vi "ErrorDescription.vi"(1 "AxisReadValues.AxisErrorCode":i16) -> (0 "ErrorDescription":string)   [LabVIEW 2020, in "SMCD14_lib.lvlib"]
uses:
  SMCD14_lib.lvlib
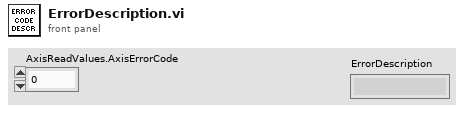
[diagram p1: front panel]
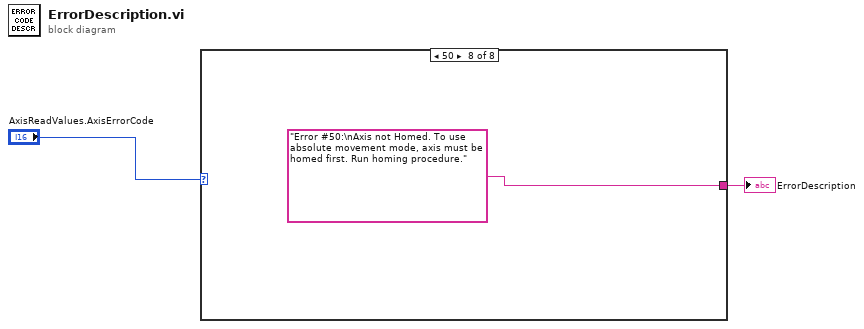
[diagram p0: block diagram]
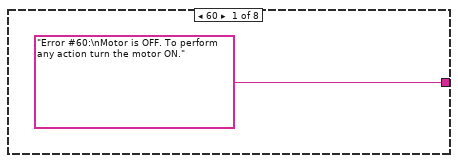
[diagram p2: hidden frame]
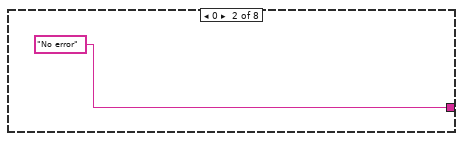
[diagram p3: hidden frame]
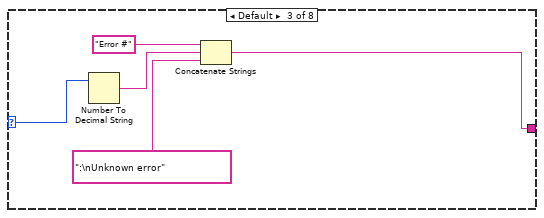
[diagram p4: hidden frame]
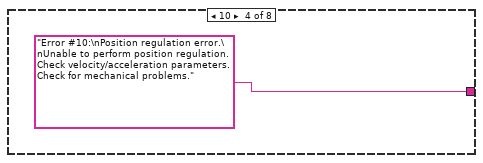
[diagram p5: hidden frame]
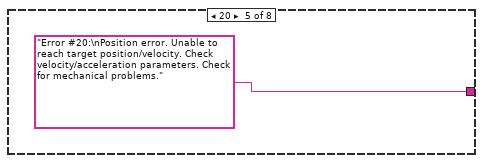
[diagram p6: hidden frame]
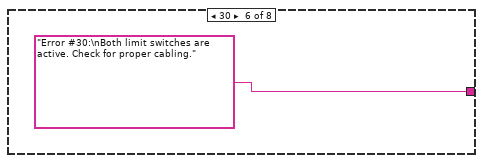
[diagram p7: hidden frame]
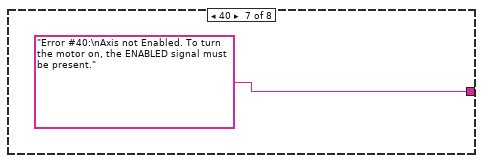
[diagram p8: hidden frame]
diagram:
  n1 = case shown="50" "AxisReadValues.AxisErrorCode" {
    selector: "AxisReadValues.AxisErrorCode" -> [_ _ w8 _ _ _ _ _]
    tunnel: ["Error #60:\nMotor is OFF. To perform any action turn the motor ON." ("ErrorDescription") "No error" ("ErrorDescription") w5 "Error #10:\nPosition regulation error.\nUnable to perform position regulation. Check velocity/acceleration parameters. Check for mechanical problems." ("ErrorDescription") "Error #20:\nPosition error. Unable to reach target position/velocity. Check velocity/acceleration parameters. Check for mechanical problems." ("ErrorDescription") "Error #30:\nBoth limit switches are active. Check for proper cabling." ("ErrorDescription") "Error #40:\nAxis not Enabled. To turn the motor on, the ENABLED signal must be present." ("ErrorDescription") "Error #50:\nAxis not Homed. To use absolute movement mode, axis must be homed first. Run homing procedure." ("ErrorDescription")] -> w1
    frame 60 {
    }
    frame 0 {
    }
    frame Default {
      n2 = Number To Decimal String(number=w8) -> (decimal integer string=w7:string)  [unwired: 1 in]
      n3 = Concatenate Strings("Error #" ("string"), w7, ":\nUnknown error" ("ErrorDescription")) -> (w5:string)
    }
    frame 10 {
    }
    frame 20 {
    }
    frame 30 {
    }
    frame 40 {
    }
    frame 50 {
    }
  }
  "ErrorDescription" <- w1
